vi "Input Data.vi"() -> ()   [LabVIEW 2013]
uses:
  qwtblvlib/TD Quantity.ctl
  <vilib>/Analysis/Matrix/Datatypes/RealMatrix.ctl
  globals.vi
  <vilib>/Utility/xml.llb/Write to XML File(string).vi
  <vilib>/Utility/xml.llb/Read From XML File(string).vi
  <vilib>/Utility/file.llb/Read From Spreadsheet File (DBL).vi
  <vilib>/Analysis/Matrix/Numeric/Conversions/Matrix To Array - RM.vi
  qwtblvlib/QWTBLVLib.lvlib
  <vilib>/Analysis/Matrix/NI_Matrix.lvlib
panel:
  out "Is Matrix?":bool
  out "Is Vector?":bool
  out "Is Scalar?":bool
  out "Is Empty?":bool
  in  "r-randomize":bool
  in  "corr-default":bool
  in  "generate wvfrm":bool
  in  "dof-fill":bool
  in  "rand-clear":bool
  in  "corr-clear":bool
  in  "dof-clear":bool
  in  "uncertainty-clear":bool
  in  "value-clear":bool
  in  "uncertainty-fill":bool
  in  "value-load CSV":bool
  in  "Q changed signal":bool
  in  "reload Q list signal":bool
  in  "reload Q signal":bool
  in  "close":bool
  in  "Quantity":T1={"Name"="", "Value"=[[1.0]], "Uncertainty"=[[1.0]], "Degrees of\nFreedom"=[[10.0]], "Correlation"=[[10.0]], "Randomized uncertainty"=[[10.0]]}
  in  "load Q":bool
  in  "save Q":bool
  in  "Q list":i32(listbox) caption="Input Quantities"
  in  "remove Q":bool
  in  "add Q":bool
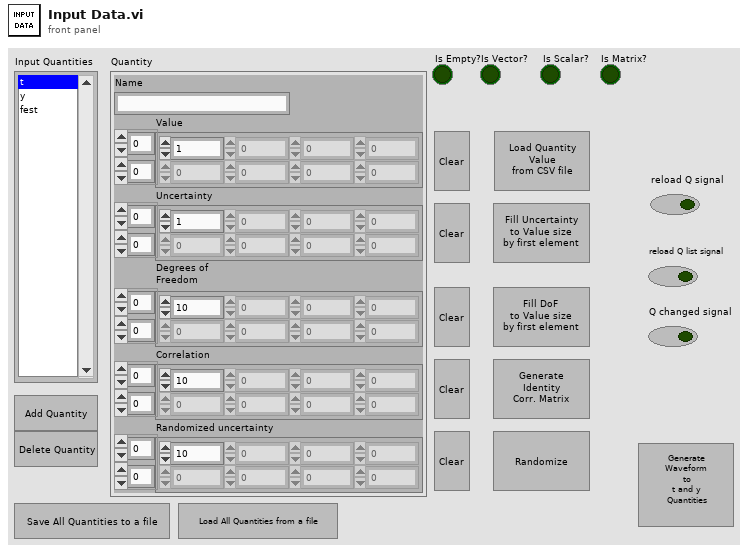
[diagram p1: front panel]
types:
  T1 = typedef "QWTBLVLib.lvlib/TD Quantity.ctl" = cluster{"Name":string, "Value":dbl[][], "Uncertainty":dbl[][], "Degrees of\nFreedom":dbl[][], "Correlation":dbl[][], "Randomized uncertainty":dbl[][]}
  T2 = typedef "NI_Matrix.lvlib/RealMatrix.ctl" = dbl[][]
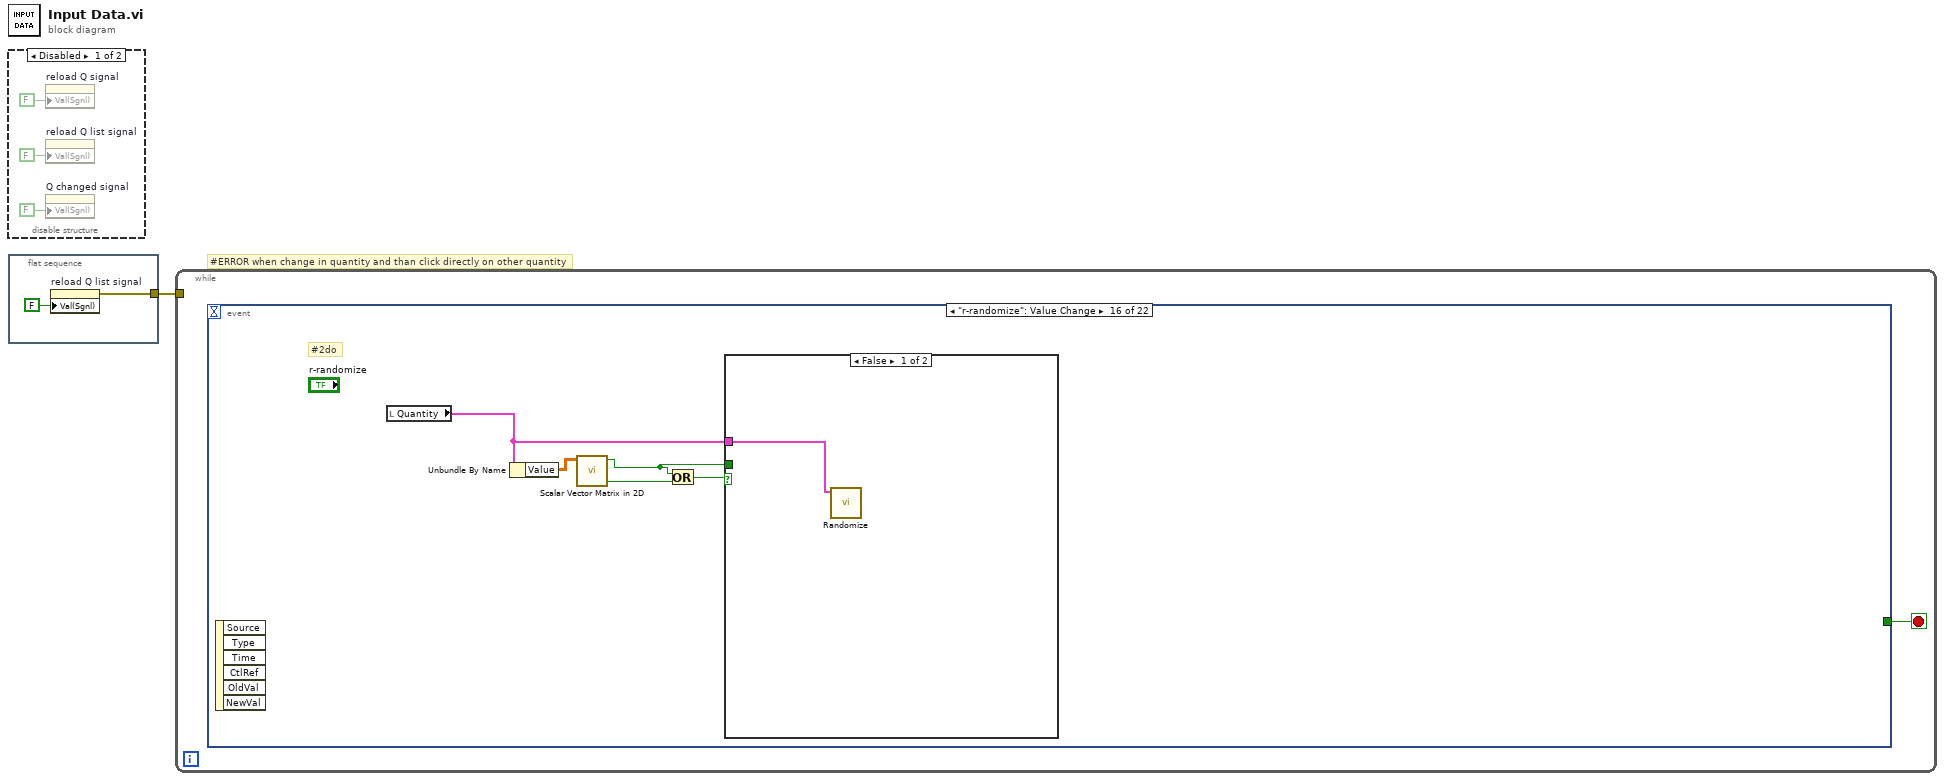
[diagram p0: block diagram]
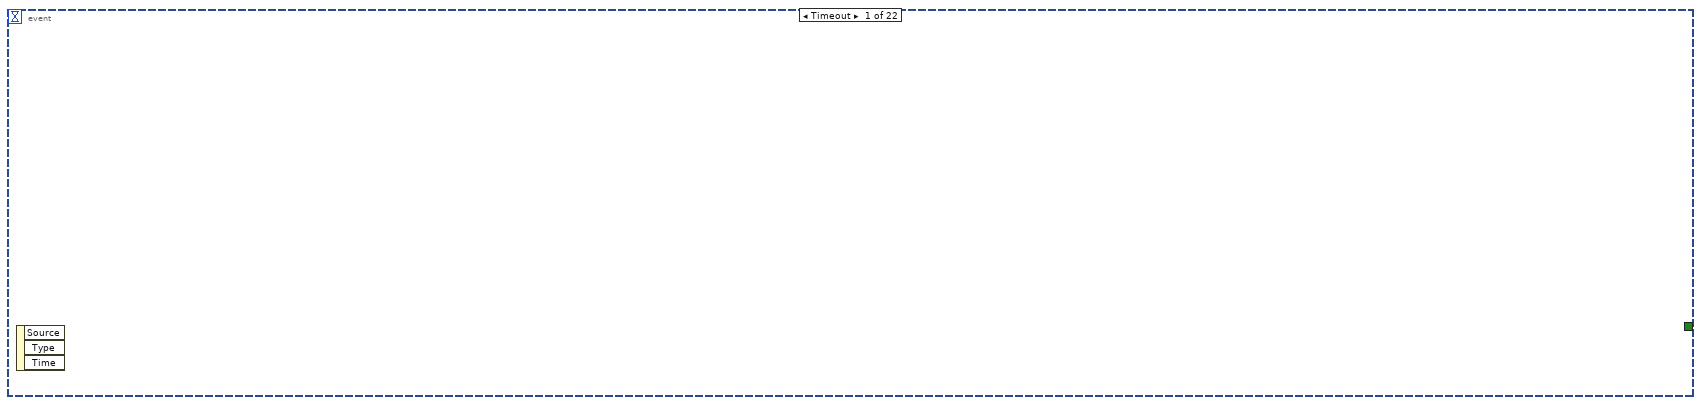
[diagram p3: hidden frame]
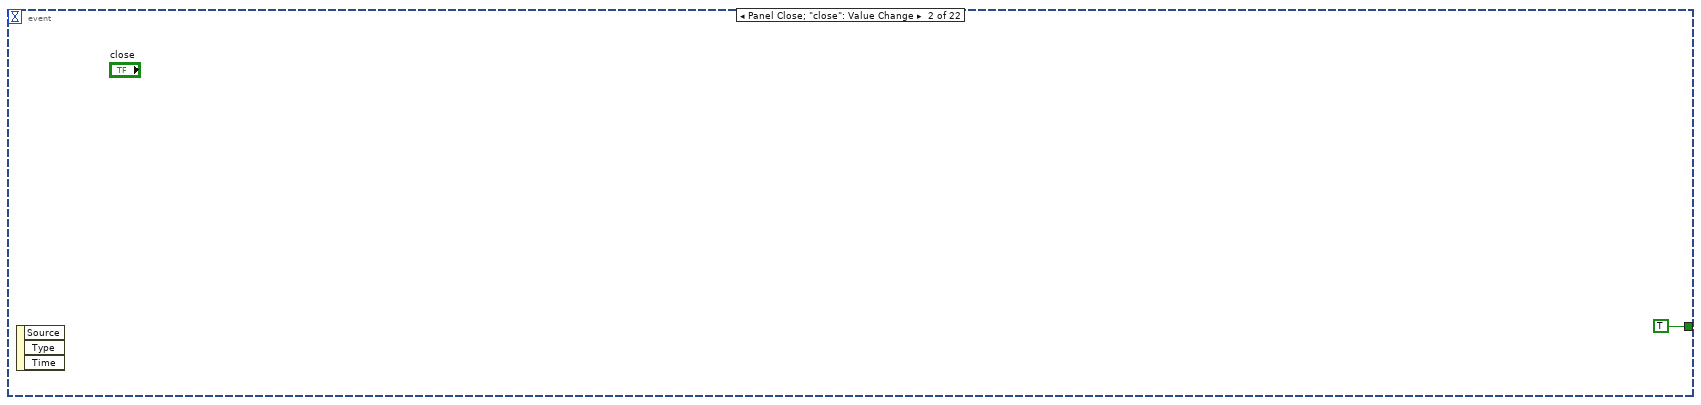
[diagram p4: hidden frame]
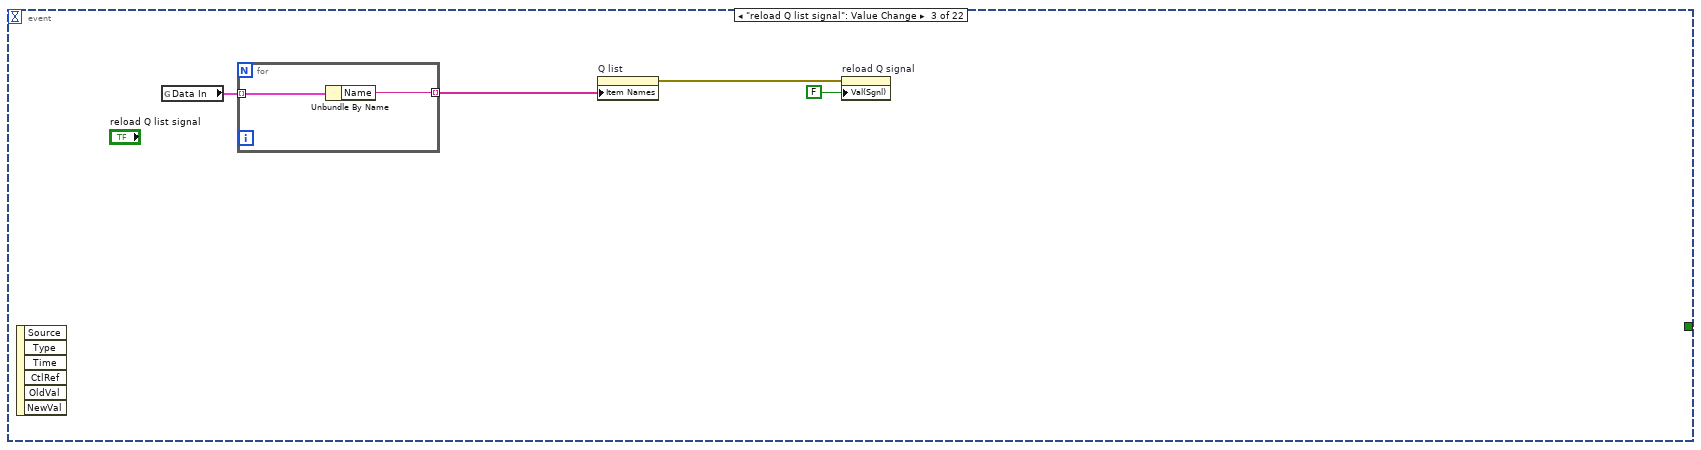
[diagram p5: hidden frame]
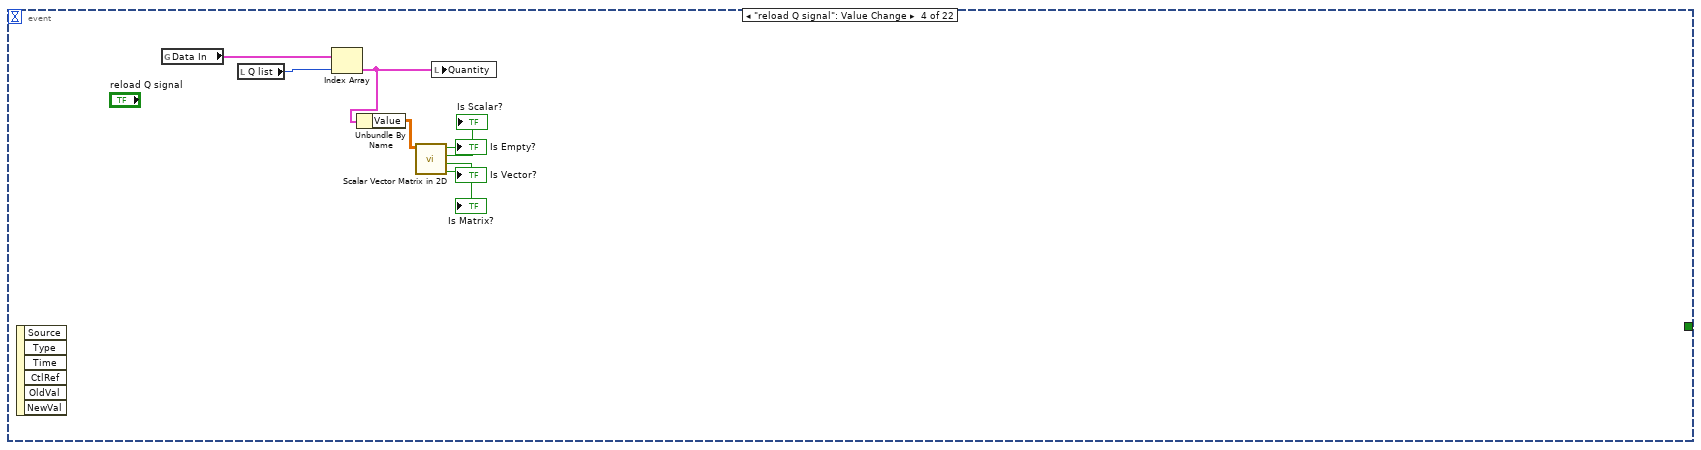
[diagram p6: hidden frame]
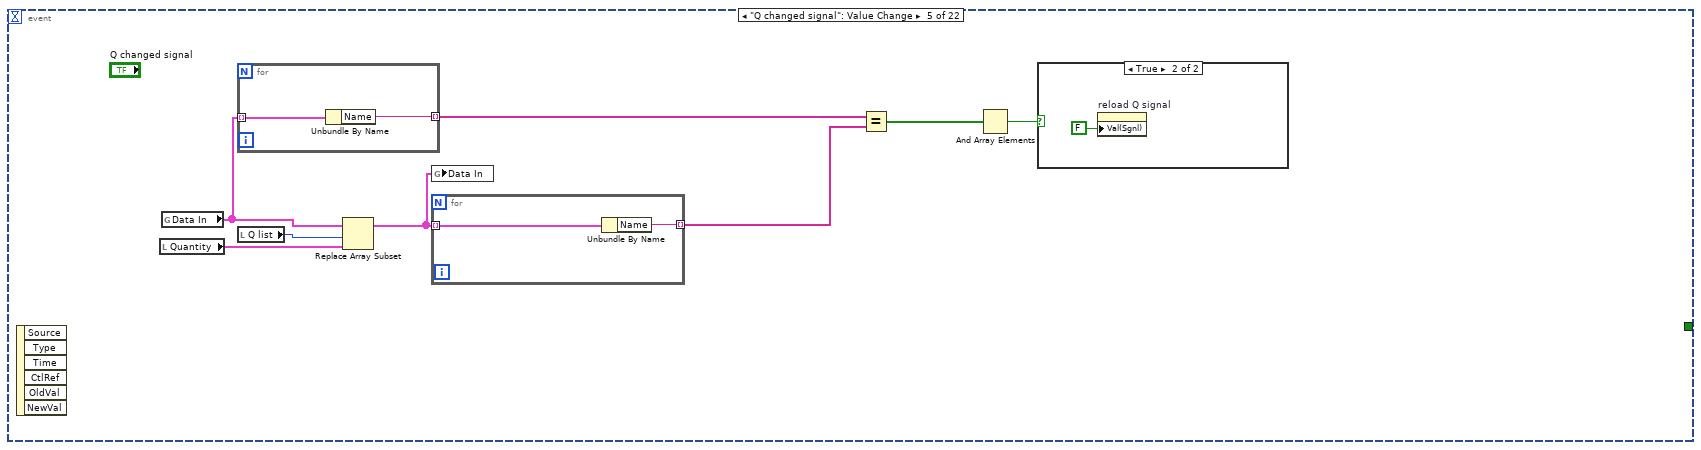
[diagram p7: hidden frame]
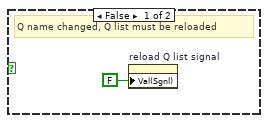
[diagram p8: hidden frame]
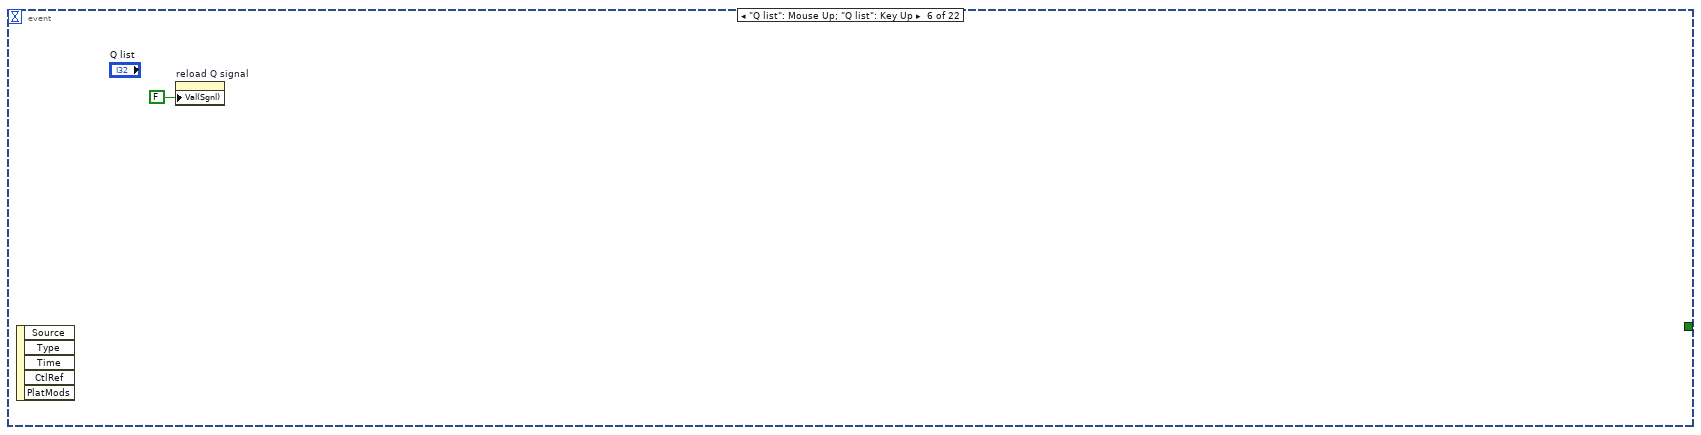
[diagram p9: hidden frame]
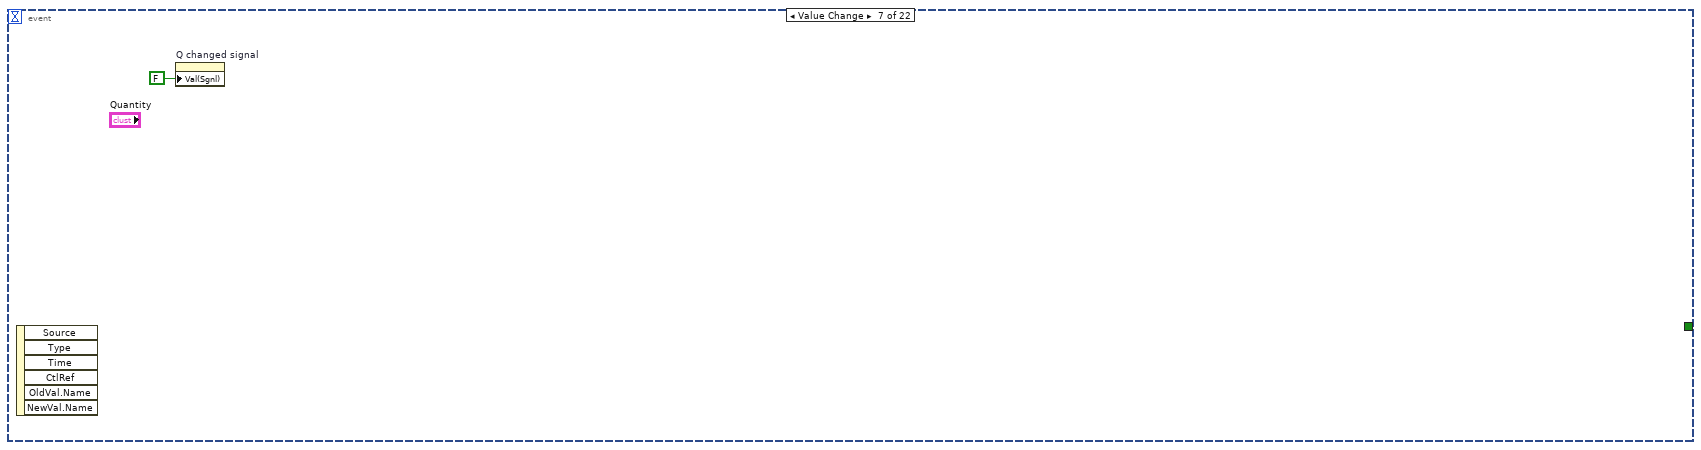
[diagram p10: hidden frame]
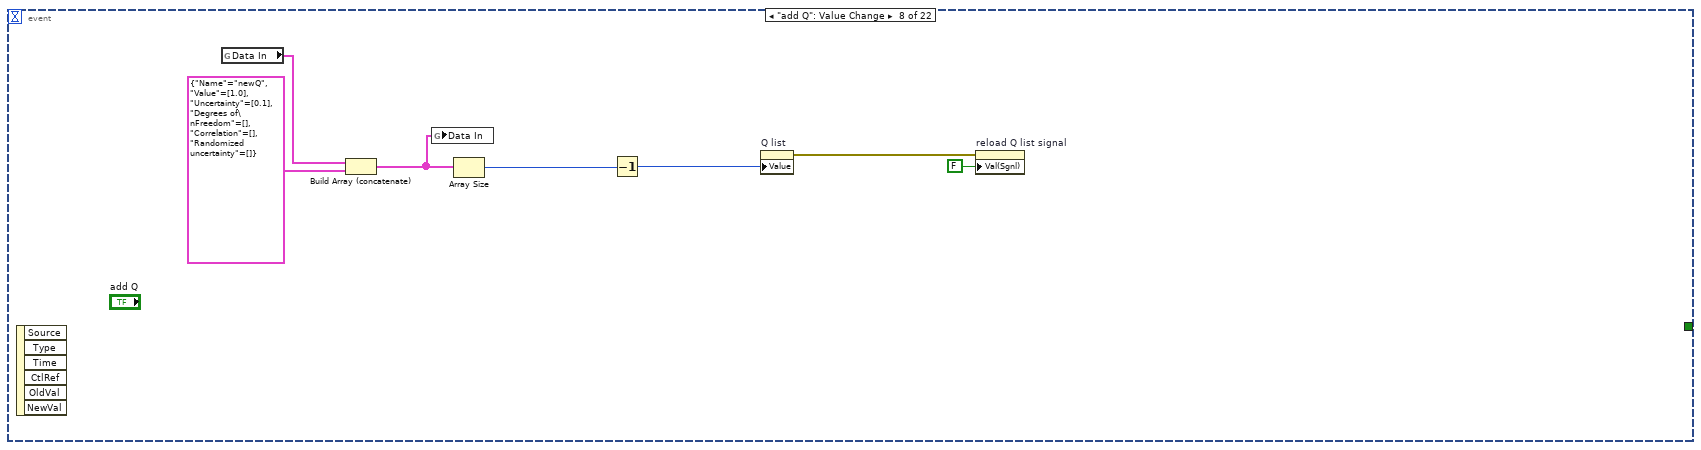
[diagram p11: hidden frame]
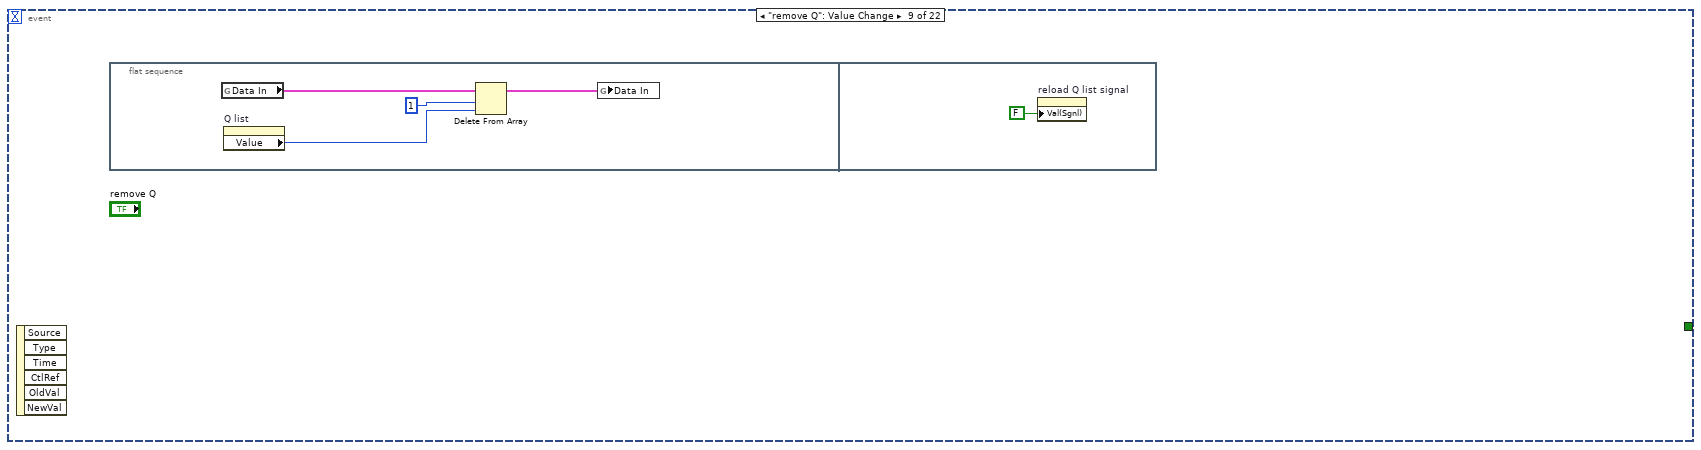
[diagram p12: hidden frame]
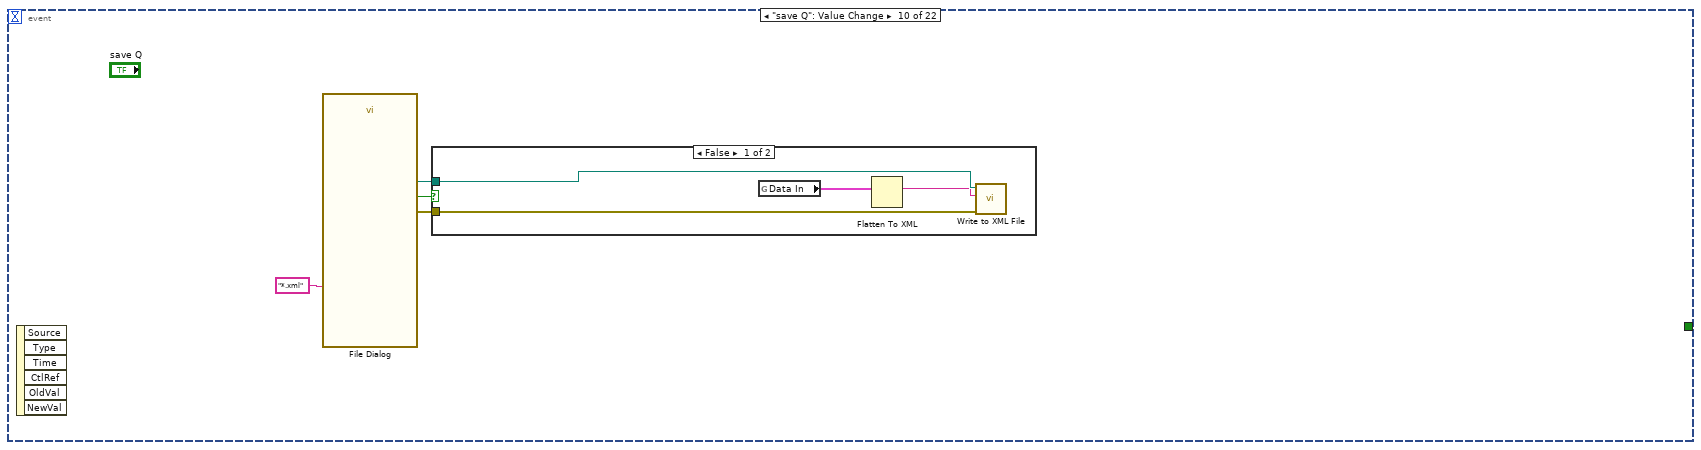
[diagram p13: hidden frame]
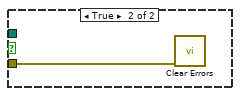
[diagram p14: hidden frame]
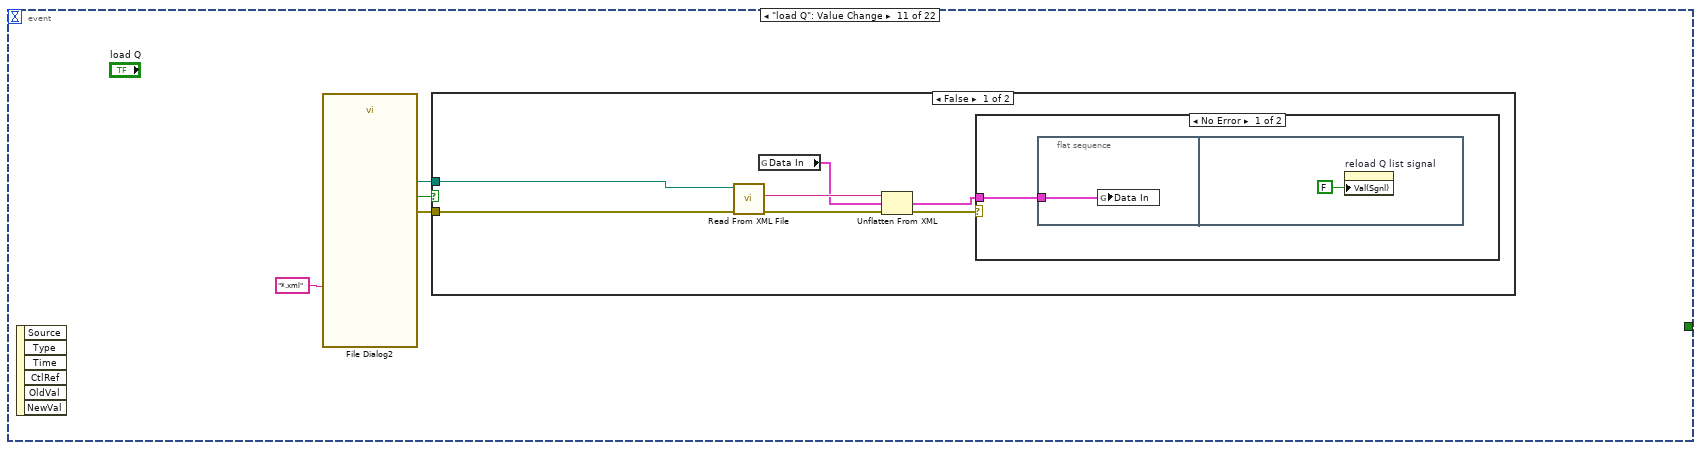
[diagram p15: hidden frame]
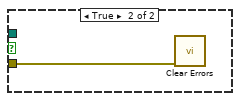
[diagram p17: hidden frame]
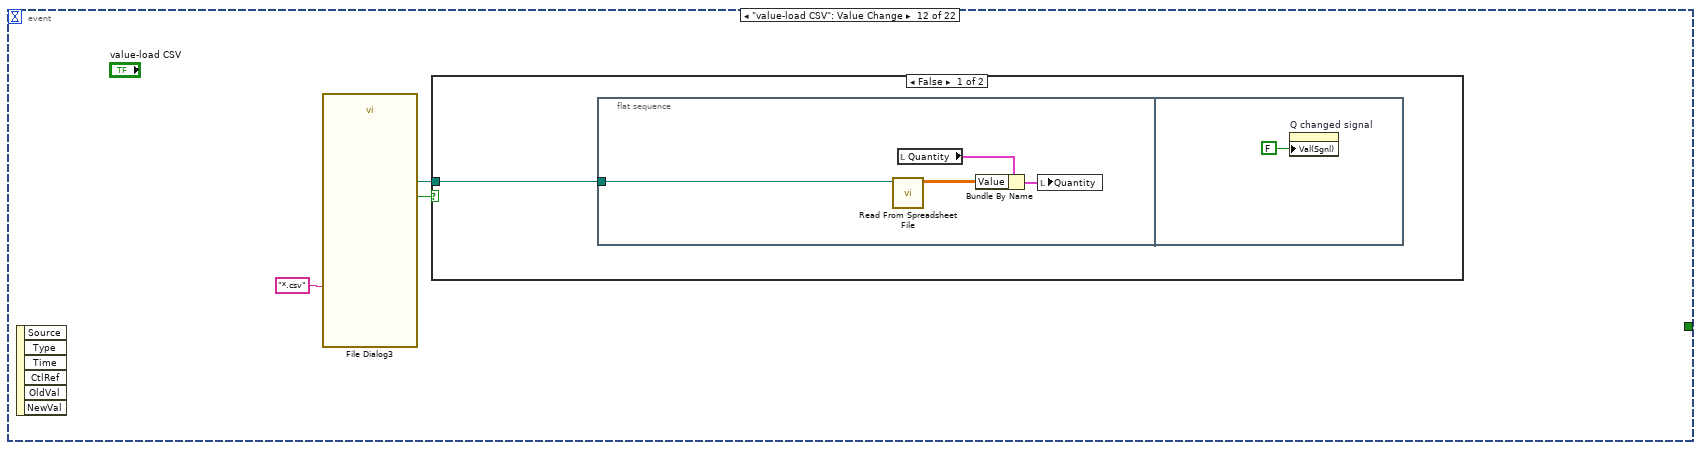
[diagram p18: hidden frame]
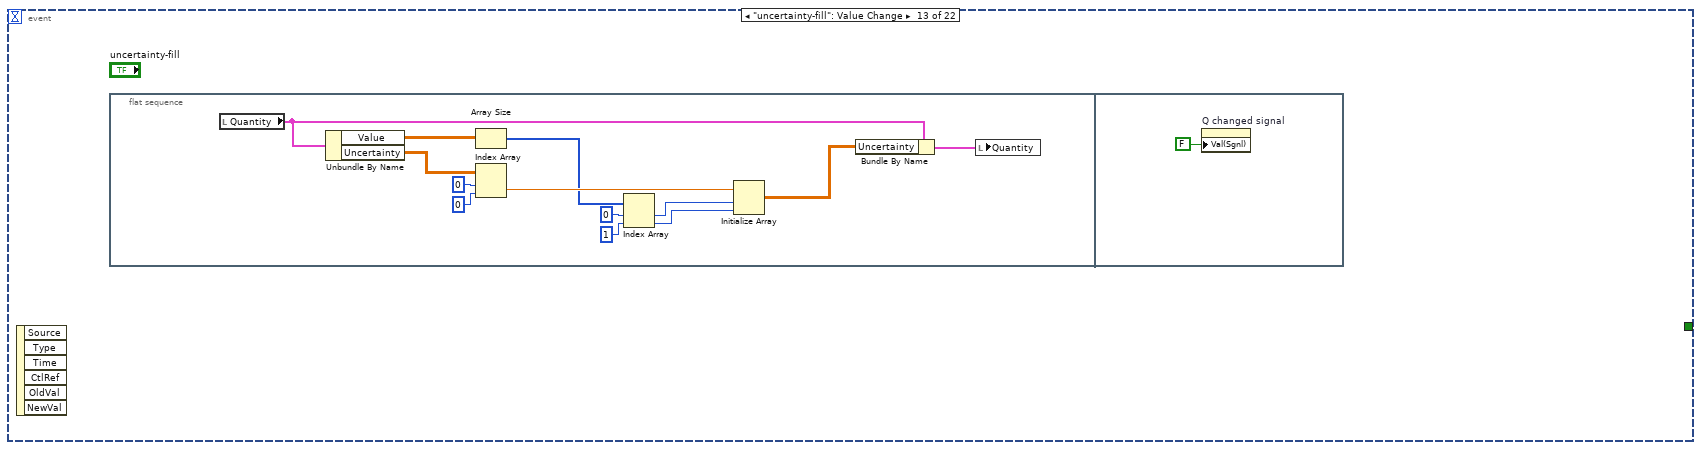
[diagram p20: hidden frame]
diagram:
  # "#ERROR when change in quantity and than click directly on other quantity"
  n1 = disable-structure shown="Disabled" {
    frame Disabled {
      n2 = property on="reload Q signal" class="Bool (strict)"("Val(Sgnl)"=FALSE ("Value (Signaling)")) -> ()  [unwired: 2 in, 2 out]
      n3 = property on="reload Q list signal" class="Bool (strict)"("Val(Sgnl)"=FALSE ("Value (Signaling)")) -> ()  [unwired: 2 in, 2 out]
      n4 = property on="Q changed signal" class="Bool (strict)"("Val(Sgnl)"=FALSE ("Value (Signaling)")) -> ()  [unwired: 2 in, 2 out]
    }
    frame Enabled {
    }
  }
  n5 = flat-sequence {
    tunnel: [w5] -> w1
    frame #0 {
      n6 = property on="reload Q list signal" class="Bool (strict)"("Val(Sgnl)"=FALSE ("Value (Signaling)")) -> (error out=w5:errorcluster)  [unwired: 2 in, 1 out]
    }
  }
  n7 = while {
    tunnel: w1 -> [_]
    stop <- w7 stop-if-true
    n8 = event shown="[15] \"r-randomize\": Value Change" {
      selector: _ -> [_ _ _ _ _ _ _ _ _ _ _ _ _ _ _ _ _ _ _ _ _ _]
      dyn-events: _ -> [_ _ _ _ _ _ _ _ _ _ _ _ _ _ _ _ _ _ _ _ _ _]
      timeout: _ -> [_ _ _ _ _ _ _ _ _ _ _ _ _ _ _ _ _ _ _ _ _ _]
      tunnel: [_ TRUE _ _ _ _ _ _ _ _ _ _ _ _ _ _ _ _ _ _ _ _] -> w7
      event Timeout {
        n9 = event-data() -> ()  [unwired: 1 in, 3 out]
      }
      event Panel Close; "close": Value Change {
        n10 = event-data() -> ()  [unwired: 1 in, 3 out]
      }
      event "reload Q list signal": Value Change {
        n11 = event-data() -> ()  [unwired: 1 in, 6 out]
        n12 = global read "globals.vi" "Data In"() -> (w11:T1[])
        n13 = for {
          tunnel: [w14] -> w10 mode=indexing
          tunnel: w11 -> [w13] mode=indexing
          n14 = Unbundle By Name(w13) -> ("Name"=w14:string)
        }
        n15 = property on="Q list" class="LstBox (strict)"("Item Names"=w10) -> (error out=w9:errorcluster)  [unwired: 2 in, 1 out]
        n16 = property on="reload Q signal" class="Bool (strict)"(error in=w9, "Val(Sgnl)"=FALSE ("Value (Signaling)")) -> ()  [unwired: 1 in, 2 out]
      }
      event "reload Q signal": Value Change {
        n17 = event-data() -> ()  [unwired: 1 in, 6 out]
        n18 = global read "globals.vi" "Data In"() -> (w22:T1[])
        n19 = local read "Q list"() -> (w21:i32)
        n20 = Index Array(array=w22, index=w21) -> (element=w20:T1)
        n21 = Unbundle By Name(w20) -> ("Value"=w19:dbl[][])
        n22 = call "Scalar Vector Matrix in 2D.vi"("2D Array"=w19) -> ("Is Matrix?"=→"Is Matrix?":bool, "Is Vector?"=→"Is Vector?":bool, "Is Scalar?"=→"Is Scalar?":bool, "Is Empty?"=→"Is Empty?":bool)  [unwired: 4 in, 3 out]
        n23 = local write "Quantity"(w20) -> ()
      }
      event "Q changed signal": Value Change {
        n24 = event-data() -> ()  [unwired: 1 in, 6 out]
        n25 = local read "Quantity"() -> (w29:T1)
        n26 = global read "globals.vi" "Data In"() -> (w28:T1[])
        n27 = for {
          tunnel: [w34] -> w26 mode=indexing
          tunnel: w28 -> [w33] mode=indexing
          n28 = Unbundle By Name(w33) -> ("Name"=w34:string)
        }
        n29 = local read "Q list"() -> (w30:i32)
        n30 = Replace Array Subset(array=w28, new element=w29, index=w30) -> (w27:T1[])
        n31 = global write "globals.vi" "Data In"(w27) -> ()
        n32 = for {
          tunnel: [w32] -> w24 mode=indexing
          tunnel: w27 -> [w31] mode=indexing
          n33 = Unbundle By Name(w31) -> ("Name"=w32:string)
        }
        n34 = Equal?(x=w26, y=w24) -> (x = y?=w23:bool[])
        n35 = And Array Elements(Boolean array=w23) -> (logical AND=w25:bool)
        n36 = case shown="True" w25 {
          frame False {
            # "Q name changed, Q list must be reloaded"
            n37 = property on="reload Q list signal" class="Bool (strict)"("Val(Sgnl)"=FALSE ("Value (Signaling)")) -> ()  [unwired: 2 in, 2 out]
          }
          frame True {
            n38 = property on="reload Q signal" class="Bool (strict)"("Val(Sgnl)"=FALSE ("Value (Signaling)")) -> ()  [unwired: 2 in, 2 out]
          }
        }
      }
      event "Q list": Mouse Up; "Q list": Key Up {
        n39 = event-data() -> ()  [unwired: 1 in, 5 out]
        n40 = property on="reload Q signal" class="Bool (strict)"("Val(Sgnl)"=FALSE ("Value (Signaling)")) -> ()  [unwired: 2 in, 2 out]
      }
      event Value Change {
        n41 = event-data() -> ()  [unwired: 1 in, 6 out]
        n42 = property on="Q changed signal" class="Bool (strict)"("Val(Sgnl)"=FALSE ("Value (Signaling)")) -> ()  [unwired: 2 in, 2 out]
      }
      event "add Q": Value Change {
        n43 = event-data() -> ()  [unwired: 1 in, 6 out]
        n44 = global read "globals.vi" "Data In"() -> (w42:T1[])
        n45 = Build Array (concatenate)(w42, T1 {"Name"="newQ", "Value"=[[1.0]], "Uncertainty"=[[0.1]], "Degrees of\nFreedom"=[], "Correlation"=[], "Randomized uncertainty"=[]} ("Quantity")) -> (w39:T1[])
        n46 = global write "globals.vi" "Data In"(w39) -> ()
        n47 = Array Size(array=w39) -> (size(s)=w45:i32)
        n48 = Decrement(x=w45) -> (x-1=w44:i32)
        n49 = property on="Q list" class="LstBox (strict)"("Value"=w44) -> (error out=w40:errorcluster)  [unwired: 2 in, 1 out]
        n50 = property on="reload Q list signal" class="Bool (strict)"(error in=w40, "Val(Sgnl)"=FALSE ("Value (Signaling)")) -> ()  [unwired: 1 in, 2 out]
      }
      event "remove Q": Value Change {
        n51 = event-data() -> ()  [unwired: 1 in, 6 out]
        n52 = flat-sequence {
          frame #0 {
            n53 = global read "globals.vi" "Data In"() -> (w47:T1[])
            n54 = property on="Q list" class="LstBox (strict)"() -> ("Value"=w48:i32)  [unwired: 2 in, 2 out]
            n55 = Delete From Array(array=w47, length=1, index=w48) -> (array with subset deleted=w46:T1[])  [unwired: 1 out]
            n56 = global write "globals.vi" "Data In"(w46) -> ()
          }
          frame #1 {
            n57 = property on="reload Q list signal" class="Bool (strict)"("Val(Sgnl)"=FALSE ("Value (Signaling)")) -> ()  [unwired: 2 in, 2 out]
          }
        }
      }
      event "save Q": Value Change {
        n58 = event-data() -> ()  [unwired: 1 in, 6 out]
        n59 = call "File Dialog"("pattern (all files)"="*.xml") -> ("selected path"=w54:path, "cancelled"=w52:bool, "error out"=w53:errorcluster)  [unwired: 11 in, 1 out]
        n60 = case shown="False" w52 {
          tunnel: w53 -> [w57 w59]
          tunnel: w54 -> [w58 _]
          frame False {
            n61 = global read "globals.vi" "Data In"() -> (w55:T1[])
            n62 = Flatten To XML(anything=w55) -> (xml string=w56:string)
            n63 = call-poly <vilib>:"Write to XML File.vi"("error in (no error)"=w57, "XML Input"=w56, "XML File Path"=w58) -> ()  [unwired: 6 in, 3 out]
          }
          frame True {
            n64 = call <vilib>:"Clear Errors.vi"("error in (no error)"=w59) -> ()  [unwired: 6 in, 1 out]
          }
        }
      }
      event "load Q": Value Change {
        n65 = event-data() -> ()  [unwired: 1 in, 6 out]
        n66 = call "File Dialog2"("pattern (all files)"="*.xml") -> ("selected path"=w63:path, "cancelled"=w61:bool, "error out"=w62:errorcluster)  [unwired: 11 in, 1 out]
        n67 = case shown="False" w61 {
          tunnel: w62 -> [w69 w74]
          tunnel: w63 -> [w70 _]
          frame False {
            n68 = call-poly <vilib>:"Read From XML File.vi"("error in (no error)"=w69, "XML File Path"=w70) -> ("error out"=w67:errorcluster, "XML Elements"=w68:string)  [unwired: 7 in, 1 out]
            n69 = global read "globals.vi" "Data In"() -> (w64:T1[])
            n70 = Unflatten From XML(xml string=w68, type=w64, error in (no error)=w67) -> (value=w65:T1[], error out=w66:errorcluster)
            n71 = case shown="No Error" w66 {
              tunnel: w65 -> [w71 _]
              frame No Error {
                n72 = flat-sequence {
                  tunnel: w71 -> [w72]
                  frame #0 {
                    n73 = global write "globals.vi" "Data In"(w72) -> ()
                  }
                  frame #1 {
                    n74 = property on="reload Q list signal" class="Bool (strict)"("Val(Sgnl)"=FALSE ("Value (Signaling)")) -> ()  [unwired: 2 in, 2 out]
                  }
                }
              }
              frame Error {
              }
            }
          }
          frame True {
            n75 = call <vilib>:"Clear Errors.vi"("error in (no error)"=w74) -> ()  [unwired: 6 in, 1 out]
          }
        }
      }
      event "value-load CSV": Value Change {
        n76 = event-data() -> ()  [unwired: 1 in, 6 out]
        n77 = call "File Dialog3"("pattern (all files)"="*.csv") -> ("selected path"=w75:path, "cancelled"=w76:bool)  [unwired: 11 in, 2 out]
        n78 = case shown="False" w76 {
          tunnel: w75 -> [w78 _]
          frame False {
            n79 = flat-sequence {
              tunnel: w78 -> [w82]
              frame #0 {
                n80 = call-poly <vilib>:"Read From Spreadsheet File.vi"("file path (dialog if empty)"=w82) -> ("all rows"=w80:dbl[][])  [unwired: 6 in, 4 out]
                n81 = local read "Quantity"() -> (w81:T1)
                n82 = Bundle By Name(cluster=w81, "Value"=w80) -> (w79:T1)
                n83 = local write "Quantity"(w79) -> ()
              }
              frame #1 {
                n84 = property on="Q changed signal" class="Bool (strict)"("Val(Sgnl)"=FALSE ("Value (Signaling)")) -> ()  [unwired: 2 in, 2 out]
              }
            }
          }
          frame True {
          }
        }
      }
      event "uncertainty-fill": Value Change {
        n85 = event-data() -> ()  [unwired: 1 in, 6 out]
        n86 = flat-sequence {
          frame #0 {
            n87 = local read "Quantity"() -> (w96:T1)
            n88 = Unbundle By Name(w96) -> ("Value"=w94:dbl[][], "Uncertainty"=w84:dbl[][])
            n89 = Array Size(array=w94) -> (size(s)=w90:i32[])
            n90 = Index Array(array=w84, index (row)=0, index (col)=0 ("disabled index (col)")) -> (element=w91:dbl)
            n91 = Index Array(array=w90, index #1=0 ("index"), index #2=1 ("index")) -> (element #1=w87:i32, element #2=w86:i32)
            n92 = Initialize Array(w91, w87, w86) -> (w85:dbl[][])
            n93 = Bundle By Name(cluster=w96, "Uncertainty"=w85) -> (w95:T1)
            n94 = local write "Quantity"(w95) -> ()
          }
          frame #1 {
            n95 = property on="Q changed signal" class="Bool (strict)"("Val(Sgnl)"=FALSE ("Value (Signaling)")) -> ()  [unwired: 2 in, 2 out]
          }
        }
      }
      event "dof-fill": Value Change {
        n96 = event-data() -> ()  [unwired: 1 in, 6 out]
        n97 = flat-sequence {
          frame #0 {
            n98 = local read "Quantity"() -> (w110:T1)
            n99 = Unbundle By Name(w110) -> ("Value"=w108:dbl[][], "Degrees of\nFreedom"=w98:dbl[][])
            n100 = Array Size(array=w108) -> (size(s)=w104:i32[])
            n101 = Index Array(array=w98, index (row)=0, index (col)=0 ("disabled index (col)")) -> (element=w105:dbl)
            n102 = Index Array(array=w104, index #1=0 ("index"), index #2=1 ("index")) -> (element #1=w101:i32, element #2=w100:i32)
            n103 = Initialize Array(w105, w101, w100) -> (w99:dbl[][])
            n104 = Bundle By Name(cluster=w110, "Degrees of\nFreedom"=w99) -> (w109:T1)
            n105 = local write "Quantity"(w109) -> ()
          }
          frame #1 {
            n106 = property on="Q changed signal" class="Bool (strict)"("Val(Sgnl)"=FALSE ("Value (Signaling)")) -> ()  [unwired: 2 in, 2 out]
          }
        }
      }
      event "corr-default": Value Change {
        n107 = event-data() -> ()  [unwired: 1 in, 6 out]
        n108 = flat-sequence {
          frame #0 {
            n109 = local read "Quantity"() -> (w118:T1)
            n110 = Unbundle By Name(w118) -> ("Value"=w116:dbl[][])
            n111 = call "Scalar Vector Matrix in 2D.vi"("2D Array"=w116) -> ("Is Matrix?"=w115:bool, "Is Empty?"=w112:bool, "Dim Max"=w113:i32, "Dimensions"=w114:i32[])  [unwired: 4 in, 3 out]
            n112 = case shown="True" w112 {
              tunnel: w118 -> [w123 w137]
              tunnel: [w122 w136] -> w117
              tunnel: w115 -> [w121 _]
              tunnel: w114 -> [w120 _]
              tunnel: w113 -> [w119 _]
              frame False {
                # "vector or matrix"
                n113 = case shown="False" w121 {
                  tunnel: w123 -> [w133 w134]
                  tunnel: [w132 w134] -> w122
                  tunnel: w120 -> [_ _]
                  tunnel: w119 -> [w124 _]
                  frame False {
                    # "vector"
                    n114 = Resize Matrix(1:w124, 2:w124, 4:T2 [] ("matrix")) -> (0:w127:T2)
                    n115 = Replace Array Subset(array=w127, new element=1.0 ("new diagonal/fill element"), index (row)=0 ("disabled index (row)"), index (col)=0 ("disabled index (col)")) -> (w126:T2)
                    n116 = call-poly <vilib>:"Matrix To Array.vi"("Real Matrix"=w126) -> ("Real 2D Array"=w125:dbl[][])
                    n117 = Bundle By Name(cluster=w133, "Correlation"=w125) -> (w132:T1)
                  }
                  frame True {
                    # "matrix"
                  }
                }
              }
              frame True {
                # "empty array"
                n118 = Bundle By Name(cluster=w137, "Correlation"=dbl[][] []) -> (w136:T1)
              }
            }
            n119 = local write "Quantity"(w117) -> ()
          }
          frame #1 {
            n120 = property on="Q changed signal" class="Bool (strict)"("Val(Sgnl)"=FALSE ("Value (Signaling)")) -> ()  [unwired: 2 in, 2 out]
          }
        }
      }
      event "r-randomize": Value Change {
        # "#2do"
        n121 = event-data() -> ()  [unwired: 1 in, 6 out]
        n122 = local read "Quantity"() -> (w139:T1)
        n123 = Unbundle By Name(w139) -> ("Value"=w143:dbl[][])
        n124 = call "Scalar Vector Matrix in 2D.vi"("2D Array"=w143) -> ("Is Matrix?"=w142:bool, "Is Empty?"=w140:bool)  [unwired: 4 in, 5 out]
        n125 = Or(x=w140, y=w142) -> (x .or. y?=w141:bool)
        n126 = case shown="False" w141 {
          tunnel: w140 -> [_ w145]
          tunnel: w139 -> [w144 _]
          frame False {
            n127 = call "Randomize.vi"("Quantity"=w144) -> ()  [unwired: 11 in]
          }
          frame True {
            n128 = case shown="False" w145 {
              frame False {
                n129 = One Button Dialog(message="Cannot do for matrix quantity.\nImplemented only for scalars or vectors.", button name ("OK")="OK") -> ()  [unwired: 1 out]
              }
              frame True {
                n130 = One Button Dialog(message="Value matrix is empty!", button name ("OK")="OK") -> ()  [unwired: 1 out]
              }
            }
          }
        }
      }
      event "value-clear": Value Change {
        n131 = event-data() -> ()  [unwired: 1 in, 6 out]
        n132 = flat-sequence {
          frame #0 {
            n133 = local read "Quantity"() -> (w152:T1)
            n134 = Bundle By Name(cluster=w152, "Value"=dbl[][] []) -> (w151:T1)
            n135 = local write "Quantity"(w151) -> ()
          }
          frame #1 {
            n136 = property on="Q changed signal" class="Bool (strict)"("Val(Sgnl)"=FALSE ("Value (Signaling)")) -> ()  [unwired: 2 in, 2 out]
          }
        }
      }
      event "uncertainty-clear": Value Change {
        n137 = event-data() -> ()  [unwired: 1 in, 6 out]
        n138 = flat-sequence {
          frame #0 {
            n139 = local read "Quantity"() -> (w156:T1)
            n140 = Bundle By Name(cluster=w156, "Uncertainty"=dbl[][] [] ("Value")) -> (w155:T1)
            n141 = local write "Quantity"(w155) -> ()
          }
          frame #1 {
            n142 = property on="Q changed signal" class="Bool (strict)"("Val(Sgnl)"=FALSE ("Value (Signaling)")) -> ()  [unwired: 2 in, 2 out]
          }
        }
      }
      event "dof-clear": Value Change {
        n143 = event-data() -> ()  [unwired: 1 in, 6 out]
        n144 = flat-sequence {
          frame #0 {
            n145 = local read "Quantity"() -> (w160:T1)
            n146 = Bundle By Name(cluster=w160, "Degrees of\nFreedom"=dbl[][] [] ("Value")) -> (w159:T1)
            n147 = local write "Quantity"(w159) -> ()
          }
          frame #1 {
            n148 = property on="Q changed signal" class="Bool (strict)"("Val(Sgnl)"=FALSE ("Value (Signaling)")) -> ()  [unwired: 2 in, 2 out]
          }
        }
      }
      event "corr-clear": Value Change {
        n149 = event-data() -> ()  [unwired: 1 in, 6 out]
        n150 = flat-sequence {
          frame #0 {
            n151 = local read "Quantity"() -> (w164:T1)
            n152 = Bundle By Name(cluster=w164, "Correlation"=dbl[][] [] ("Value")) -> (w163:T1)
            n153 = local write "Quantity"(w163) -> ()
          }
          frame #1 {
            n154 = property on="Q changed signal" class="Bool (strict)"("Val(Sgnl)"=FALSE ("Value (Signaling)")) -> ()  [unwired: 2 in, 2 out]
          }
        }
      }
      event "rand-clear": Value Change {
        n155 = event-data() -> ()  [unwired: 1 in, 6 out]
        n156 = flat-sequence {
          frame #0 {
            n157 = local read "Quantity"() -> (w168:T1)
            n158 = Bundle By Name(cluster=w168, "Randomized uncertainty"=dbl[][] [] ("Value")) -> (w167:T1)
            n159 = local write "Quantity"(w167) -> ()
          }
          frame #1 {
            n160 = property on="Q changed signal" class="Bool (strict)"("Val(Sgnl)"=FALSE ("Value (Signaling)")) -> ()  [unwired: 2 in, 2 out]
          }
        }
      }
      event "generate wvfrm": Value Change {
        n161 = event-data() -> ()  [unwired: 1 in, 6 out]
        n162 = call "generate wvfrm.vi"() -> ("error out"=w172:errorcluster, "waveform"=w170:dbl[], "time series"=w171:dbl[], "canceled?"=w173:bool)  [unwired: 8 in]
        n163 = case shown="False" w173 {
          tunnel: w172 -> [w176 _]
          tunnel: w171 -> [w175 _]
          tunnel: w170 -> [w174 _]
          frame False {
            # "not canceled"
            n164 = case shown="No Error" w176 {
              tunnel: w175 -> [w185 _]
              tunnel: w174 -> [w181 _]
              frame No Error {
                w179 = T1 {"Name"="", "Value"=[], "Uncertainty"=[], "Degrees of\nFreedom"=[], "Correlation"=[], "Randomized uncertainty"=[]} ("Quantity")
                n165 = Build Array(w185) -> (w184:dbl[][])
                n166 = Build Array(w181) -> (w180:dbl[][])
                n167 = Bundle By Name(cluster=w179, "Name"="t", "Value"=w184) -> (w177:T1)
                n168 = Bundle By Name(cluster=w179, "Name"="y", "Value"=w180) -> (w178:T1)
                n169 = global read "globals.vi" "Data In"() -> (w189:T1[])
                n170 = Build Array (concatenate)(w189, w177, w178) -> (w186:T1[])
                n171 = global write "globals.vi" "Data In"(w186) -> ()
                n172 = Array Size(array=w186) -> (size(s)=w191:i32)
                n173 = Decrement(x=w191) -> (x-1=w190:i32)
                n174 = property on="Q list" class="LstBox (strict)"("Value"=w190) -> (error out=w187:errorcluster)  [unwired: 2 in, 1 out]
                n175 = property on="reload Q list signal" class="Bool (strict)"(error in=w187, "Val(Sgnl)"=FALSE ("Value (Signaling)")) -> ()  [unwired: 1 in, 2 out]
              }
              frame Error {
              }
            }
          }
          frame True {
          }
        }
      }
    }
  }
